vi "ChangeMode.vi"(0 "reference in":refnum<class "SecuritySystem.lvclass">, 2 "RoomName":string, 3 "Security Mode":T1, 5 "Error In":errorcluster) -> (14 "reference out":refnum<class "SecuritySystem.lvclass">, 19 "Error Out":errorcluster)   [LabVIEW 2024, in "SecuritySystem.lvclass"]
doc: "Change all security devices inside a desired room to one of the below:\n- Aggresive\n- Defensive\n- Balanced"
uses:
  SecuritySystem.lvclass
  Security Mode.ctl
  House/Room_class/Room.lvclass
  Devices/Security_class/Security.lvclass
panel:
  # "Connector Pane"
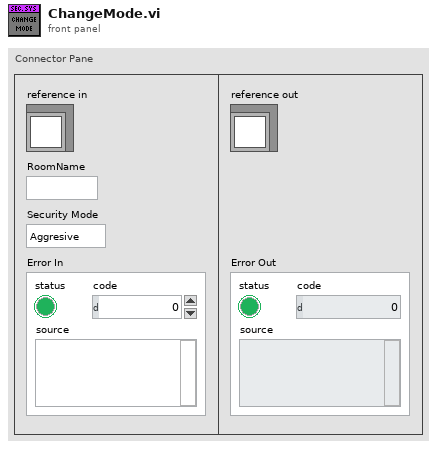
[diagram p1: front panel]
types:
  T1 = typedef "SecuritySystem.lvclass/Security Mode.ctl" = enum16{"Aggresive", "Defensive", "Balanced"}
  T2 = typedef "SecuritySystem.lvclass/ObjectAttributes.ctl" = cluster{"Rooms":T3}
  T3 = typedef "Rooms Map.ctl" = map{string, refnum<class "Room.lvclass">}
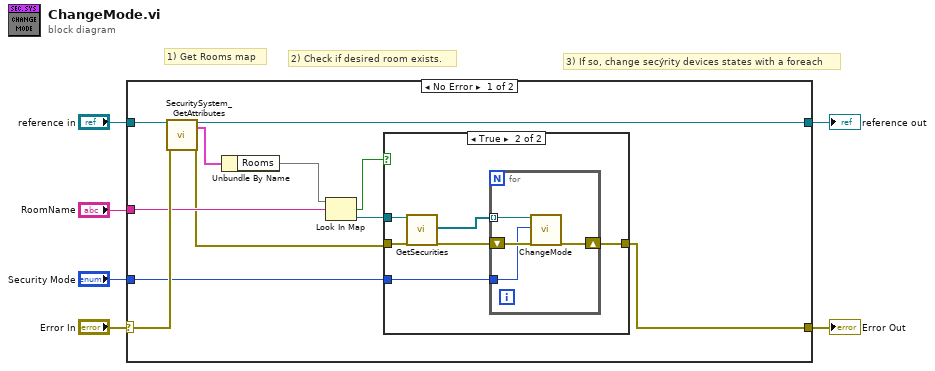
[diagram p0: block diagram]
diagram:
  # "3) If so, change secýrity devices states with a foreach"
  # "2) Check if desired room exists."
  # "1) Get Rooms map"
  n1 = case shown="No Error" "Error In" {
    selector: "Error In" -> [w17 w30]
    tunnel: [w7 w30] -> w5
    tunnel: [w14 w29] -> w3
    tunnel: "reference in" -> [w15 w29]
    tunnel: "RoomName" -> [w12 _]
    tunnel: "Security Mode" -> [w8 _]
    frame No Error {
      n2 = call "SecuritySystem_GetAttributes.vi"("reference in"=w15, "Error In"=w17) -> ("reference out"=w14:refnum<class "SecuritySystem.lvclass">, "Data"=w16:T2, "Error Out"=w9:errorcluster)  [unwired: 14 in, 1 out]
      n3 = Unbundle By Name(w16) -> ("Rooms"=w13:T3)
      n4 = Look In Map(map=w13, key=w12) -> (key not found?=w11:bool, value=w10:refnum<class "Room.lvclass">)  [unwired: 1 in]
      n5 = case shown="True" w11 {
        tunnel: w10 -> [_ w24]
        tunnel: w9 -> [w18 w23]
        tunnel: w8 -> [_ w20]
        tunnel: [w18 w19] -> w7
        frame False {
        }
        frame True {
          n6 = call-dynamic "GetSecurities.vi"("reference in"=w24, "Error In"=w23) -> ("Securities"=w21:refnum<class "Security.lvclass">[], "Error Out"=w22:errorcluster)  [unwired: 15 in, 1 out]
          n7 = for {
            tunnel: w21 -> [w27] mode=indexing
            tunnel: w20 -> [w26]
            shift-right: [w25] -> w19
            shift-left: w22 -> [w28]
            n8 = call-dynamic "ChangeMode.vi"("reference in"=w27, "Security Mode"=w26, "Error In"=w28) -> ("Error Out"=w25:errorcluster)  [unwired: 15 in, 1 out]
          }
        }
      }
    }
    frame Error {
    }
  }
  "Error Out" <- w5
  "reference out" <- w3
